vi "resonant.piezo.config.vi"() -> (3 "appended array":dbl[][](array[numeric]))   [LabVIEW 2012]
uses:
  GFG/GFGnumericGet.vi
  GFG/GFGbooleanGet.vi
  GFG/GFG library.lvlib
panel:
  out "pockels cell control":dbl[](graph)
  out "piezo control":dbl[](graph)
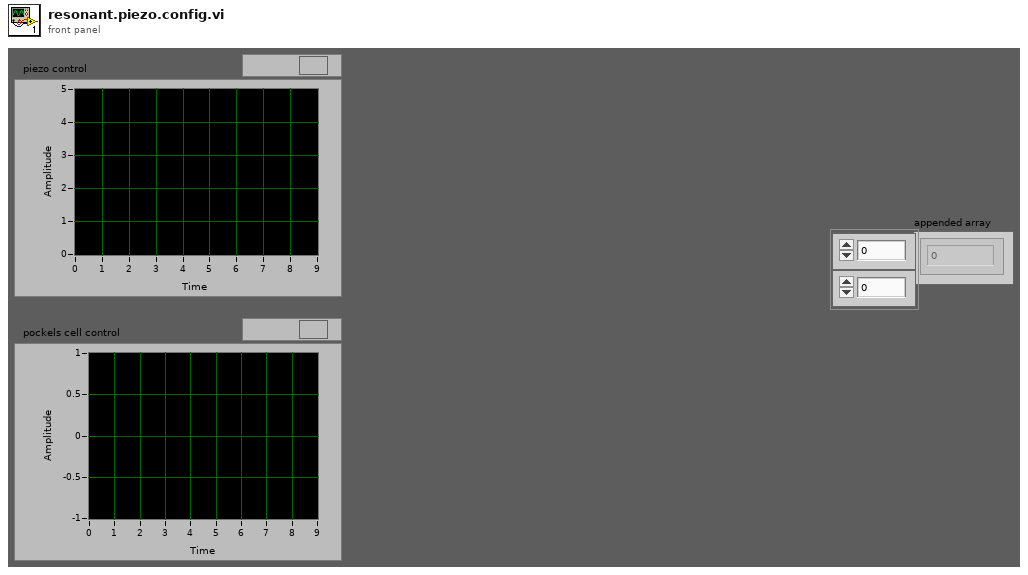
[diagram p1: front panel]
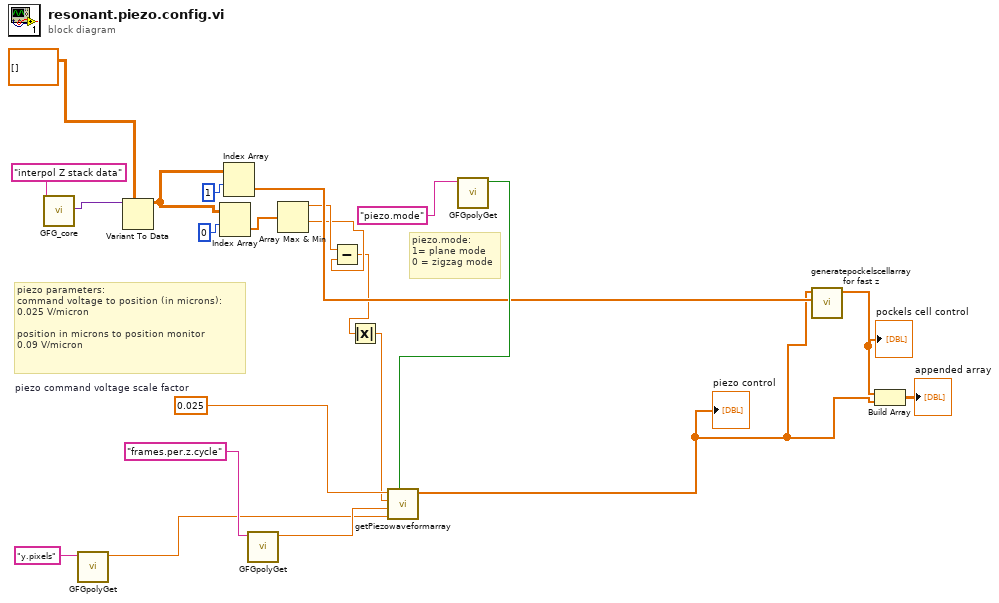
[diagram p0: block diagram]
diagram:
  w22 = 0.025  # piezo command voltage scale factor
  # "piezo.mode: \n1= plane mode\n0 = zigzag mode"
  # "piezo parameters:\ncommand voltage to position (in microns):\n0.025 V/micron\n\nposition in microns to position monitor\n0.09 V/micron"
  n1 = call "GFG_core.vi"("Variable Name in"="interpol Z stack data") -> ("Variant Out"=w17:variant)  [unwired: 12 in, 6 out]
  n2 = call-poly "GFGpolyGet.vi"("Variable Name in"="y.pixels") -> ("Numeric"=w3:dbl)  [unwired: 9 in, 1 out]
  n3 = Variant To Data(type=dbl[][] [] ("Interpolated Data"), Variant=w17) -> (data=w14:dbl[][])  [unwired: 1 in, 1 out]
  n4 = Index Array(array=w14, index (row)=0 ("disabled index (col)")) -> (element=w13:dbl[])  [unwired: 1 in]
  n5 = Index Array(array=w14, index (row)=1 ("disabled index (col)")) -> (element=w15:dbl[])  [unwired: 1 in]
  n6 = call-poly "GFGpolyGet.vi"("Variable Name in"="frames.per.z.cycle" ("Tag in")) -> ("Numeric"=w7:dbl)  [unwired: 9 in, 1 out]
  n7 = Array Max & Min(array=w13) -> (max value=w12:dbl, min value=w11:dbl)  [unwired: 2 out]
  n8 = Subtract(x=w12, y=w11) -> (x-y=w10:dbl)
  n9 = Absolute Value(x=w10) -> (abs(x)=w9:dbl)
  n10 = call-poly "GFGpolyGet.vi"("Variable Name in"="piezo.mode" ("Tag in")) -> ("Boolean"=w19:bool)  [unwired: 10 in]
  n11 = call "getPiezowaveformarray.vi"("planes or zigzag"=w19, "pixel.num"=w3, "frames.per.z.cycle"=w7, "total.z.distance"=w9, "piezo scale factor"=w22) -> ("Array"=w4:dbl[])  [unwired: 6 in]
  "piezo control" <- w4
  n12 = call "generatepockelscellarray for fast z.vi"("interpolated pockels cell data"=w15, "piezo control"=w4) -> ("pockelscellarray"=w18:dbl[])  [unwired: 9 in]
  "pockels cell control" <- w18
  n13 = Build Array(w18, w4) -> (→"appended array":dbl[][])
